vi "plot theory.vi"() -> ()   [LabVIEW 2016]
uses:
  <vilib>/Utility/file.llb/Write Delimited Spreadsheet (DBL).vi
panel:
  in  "color scale":u32[](array[colorbox])=[16711680, 16772608, 6618880, 3381759, 16860, 10420479]
  in  "length 2":i32=200
  in  "index 2":i32
  out "Intensity Graph 13":dbl[][](graph)
  in  "file path (dialog if empty)":path=path "C:/Users/ansom/OneDrive/Pascal Electron Bunching/Figures/Fig 4_new/DMRG stuff/trion_from labview.txt"
  out "Array 2":dbl[][](array[numeric])
  in  "DMRG #":i32=226
  in  "file (use dialog) 4":path=path "C:/Users/ansom/OneDrive/Pascal Electron Bunching/Figures/Fig 4_new/DMRG stuff/trion.txt"
  in  "length":i32=1000
  in  "index":i32
  out "input G":cluster{dbl[], dbl[]}[](graph)=[{[0.01, 0.02, 0.03, 0.04, 0.05, 0.060000000000000005, 0.06999999999999999, 0.08, 0.09, 0.09999999999999999, 0.11, 0.12, 0.13, 0.14, 0.15000000000000002, 0.16, 0.17, 0.18000000000000002, 0.19, 0.2, 0.21000000000000002, 0.22, 0.23, 0.24000000000000002, 0.25, 0.26, 0.27, 0.28, 0.29000000000000004, 0.3, 0.31, 0.32, 0.33, 0.34, 0.35000000000000003, 0.36000000000000004, 0.37, 0.38, 0.39, 0.4, 0.41000000000000003, 0.42000000000000004, 0.43, 0.44, 0.45, 0.46, 0.47000000000000003, 0.48000000000000004, 0.49, 0.5, 0.51, 0.52, 0.53, 0.54, 0.55, 0.56, 0.5700000000000001, 0.5800000000000001, 0.59, 0.6, 0.61, 0.62, 0.63, 0.64, 0.65, 0.66, 0.67, 0.68, 0.6900000000000001, 0.7000000000000001, 0.7100000000000001, 0.72, 0.73, 0.74, 0.75, 0.76, 0.77, 0.78, 0.79, 0.8, 0.81, 0.8200000000000001, 0.8300000000000001, 0.8400000000000001, 0.85, 0.86, 0.87, 0.88, 0.89, 0.9, 0.91, 0.92, 0.93, 0.9400000000000001, 0.9500000000000001, 0.9600000000000001, 0.97, 0.98, 0.99, 1.0, 1.01, 1.02, 1.03, 1.04, 1.05, 1.06, 1.07, 1.08, 1.09, 1.1, 1.11, 1.12, 1.1300000000000001, 1.1400000000000001, 1.1500000000000001, 1.1600000000000001, 1.17, 1.18, 1.19, 1.2, 1.21, 1.22, 1.23, 1.24, 1.25, 1.26, 1.27, 1.28, 1.29, 1.3, 1.31, 1.32, 1.33, 1.34, 1.35, 1.36, 1.37, 1.3800000000000001, 1.3900000000000001, 1.4000000000000001, 1.4100000000000001, 1.42, 1.43, 1.44, 1.45, 1.46, 1.47, 1.48, 1.49, 1.5, 1.51, 1.52, 1.53, 1.54, 1.55, 1.56, 1.57, 1.58, 1.59, 1.6, 1.61, 1.62, 1.6300000000000001, 1.6400000000000001, 1.6500000000000001, 1.6600000000000001, 1.6700000000000002, 1.68, 1.69, 1.7, 1.71, 1.72, 1.73, 1.74, 1.75, 1.76, 1.77, 1.78, 1.79, 1.8, 1.81, 1.82, 1.83, 1.84, 1.85, 1.86, 1.87, 1.8800000000000001, 1.8900000000000001, 1.9000000000000001, 1.9100000000000001, 1.9200000000000002, 1.93, 1.94, 1.95, 1.96, 1.97, 1.98, 1.99, 2.0], [0.0, 2.8179258963930954e-06, 5.865517131435599e-06, 1.1115444670828347e-05, 2.013415466013697e-05, 3.564578593329415e-05, 6.231356475073917e-05, 0.00010817567243315048, 0.0001870443462831501, 0.00032266888951518836, 0.0005559253396610961, 0.0009570334248864857, 0.0016466138487119166, 0.0028317168787741144, 0.004867094665031302, 0.008358909082529469, 0.014338061316041076, 0.02454336456201635, 0.04186555650718952, 0.07099477071552311, 0.1192181455270459, 0.19702751476009608, 0.31754465261583664, 0.4929918087827873, 0.7270707427374825, 1.0068315493607645, 1.303870994089269, 1.5898503592803936, 1.8542059202275674, 2.107927138772979, 2.372565955700939, 2.663658895477296, 2.978024236296329, 3.2945575894029333, 3.5907595763609583, 3.8607032966795023, 4.118417825912882, 4.386736502532661, 4.681005344958576, 4.997139339821397, 5.313617926593991, 5.608742028148086, 5.878098240348298, 6.136917865879712, 6.408381089034445, 6.707415756579491, 7.0295138846981375, 7.354050575014656, 7.662532325724841, 7.9559972758691035, 8.257068268102014, 8.59832499790761, 9.005858750273989, 9.485865728196863, 10.022010605260363, 10.585071760757913, 11.147313172231405, 11.695472331539898, 12.236800322485264, 12.79040913714259, 13.368853196684928, 13.96718630472856, 14.567363112985483, 15.15074818722707, 15.710997225632449, 16.26010468106789, 16.81951113752647, 17.40214872439687, 18.002767315246018, 18.60335954680593, 19.185992790268575, 19.745628904993918, 20.295452701683242, 20.85711245892441, 21.442832225062357, 22.046765008795422, 22.651313809011008, 23.240359487686586, 23.812234669482113, 24.38480624265897, 24.985518789665473, 25.634311044565536, 26.335976422740604, 27.085078807164205, 27.87323297330553, 28.692655259186335, 29.535612303041997, 30.392470291093304, 31.253112586227456, 32.11126213406538, 32.96669782438915, 33.823190913007124, 34.68503172743494, 35.55364233198232, 36.42553936546845, 37.29469772847206, 38.1576422255595, 39.015959727230076, 39.87442706067657, 40.73777794207555, 41.607477793911414, 42.479987901448624, 43.34947542419982, 44.21295855685387, 45.07258580489307, 45.9336602171978, 46.801526677239856, 47.67856262350638, 48.562979328968716, 49.452307104798635, 50.34919525380985, 51.264151190587604, 52.213679224779575, 53.21569295203033, 54.281404489557396, 55.40545289638095, 56.56294069425582, 57.72071321658015, 58.85736648074177, 59.97509976423845, 61.0945414605609, 62.237597573001054, 63.41005940897371, 64.59594439068273, 65.76911868877475, 66.9138986023004, 68.03666579771638, 69.16034526404309, 70.30725646245965, 71.48241599680148, 72.66905548648172, 73.8413370460884, 74.98496084644341, 76.1078700133423, 77.23376206365978, 78.38468495970822, 79.56489646936996, 80.75760780281024, 81.93892390590176, 83.09878006001364, 84.25127138493237, 85.4279730030069, 86.66068759066243, 87.96488912029083, 89.33334009472996, 90.74260884461259, 92.16574915118754, 93.58379408866665, 94.99404366324039, 96.40873804301812, 97.84163247726151, 99.29453862986917, 100.75605837577758, 102.21000947974164, 103.6457662539617, 105.06663578596623, 106.48846757504609, 107.92641937203824, 109.38245382309192, 110.84522457621912, 112.2989725664384, 113.7339654899229, 115.15460251908631, 116.57723208042141, 118.01649951245584, 119.47342872833094, 120.93610771377155, 122.38886223587953, 123.82265420342671, 125.24283755310711, 126.66611460936745, 128.1065090941953, 129.56404604963117, 131.02622118449602, 132.47737417640826, 133.9090314886612, 135.32721123994423, 136.7484139594865, 138.18516151830661, 139.63509629879908, 141.08280857857633, 142.50881111150676, 143.89904436452576, 145.2507726450103, 146.567316973192, 147.8447583157048, 149.06680014188356, 150.21556039701025, 151.28537528193894, 152.2847286798789, 153.22664057547803, 154.11777948305541, 154.9551366322349, 155.72976866205235, 156.43200642589352, 157.05608678065863, 157.60563194109096, 158.09445966431034, 158.53561617308696, 158.92790708641883]}, ...(100 in all)]
  in  "mu":path=path "C:/Users/ansom/OneDrive/Pascal Electron Bunching/Figures/Fig 3_new/mathematica/mu.txt"
  in  "G":path=path "C:/Users/ansom/OneDrive/Pascal Electron Bunching/Figures/Fig 3_new/mathematica/Gsteps_g=1"
  in  "Numeric 2":i32=100
  in  "Numeric":i32=360
  out "Intensity Graph 12":dbl[][](graph)
  out "Array":dbl[][](array[numeric])
  in  "file (use dialog)":path=path "C:/Users/ansom/OneDrive/Pascal Electron Bunching/Figures/Fig 3_new/mathematica/ModeldGdE"
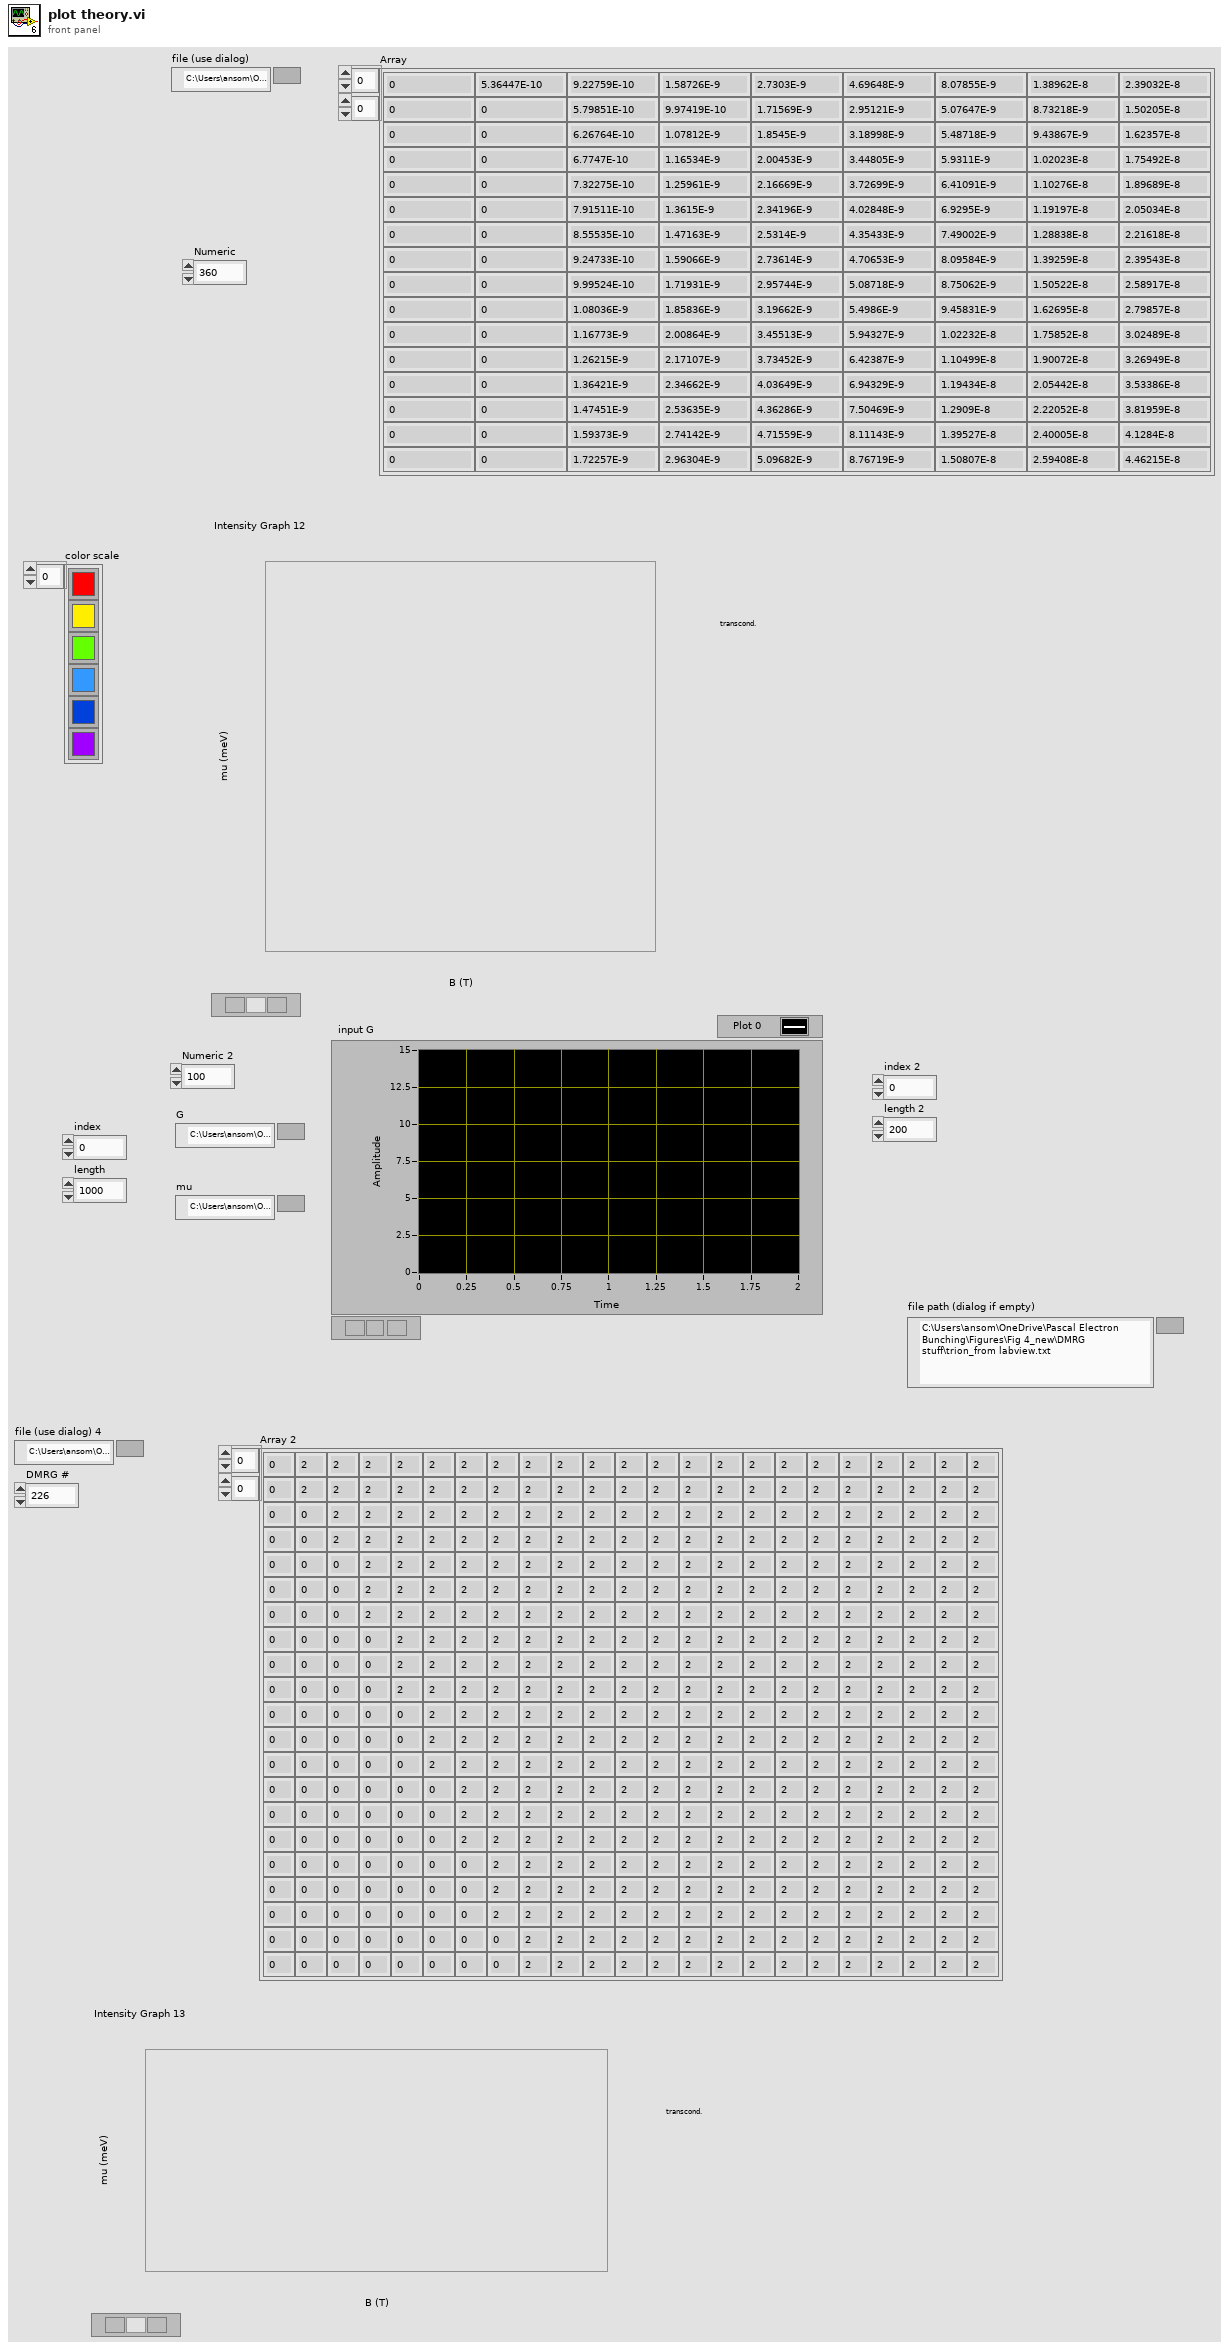
[diagram p1: front panel]
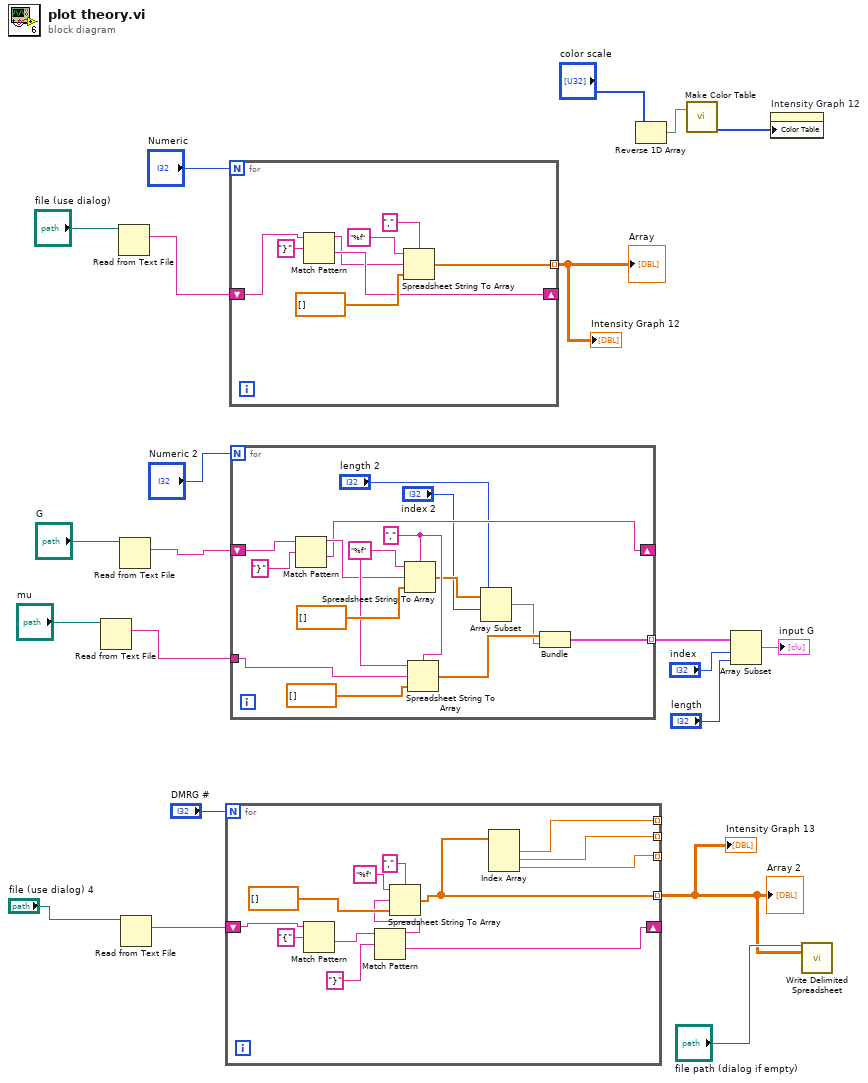
[diagram p0: block diagram]
diagram:
  n1 = Read from Text File(file (use dialog)="mu") -> (text=w14:string)  [unwired: 3 in, 3 out]
  n2 = Read from Text File(file (use dialog)="file (use dialog)") -> (text=w20:string)  [unwired: 3 in, 3 out]
  n3 = Read from Text File(file (use dialog)="G") -> (text=w13:string)  [unwired: 3 in, 3 out]
  n4 = Read from Text File(file (use dialog)="file (use dialog) 4") -> (text=w7:string)  [unwired: 3 in, 3 out]
  n5 = for {
    N: "DMRG #" -> [_]
    shift-right: [w26] -> _
    shift-left: w7 -> [w33]
    tunnel: [w25] -> w4 mode=indexing
    tunnel: [w24] -> _ mode=indexing
    tunnel: [w23] -> _ mode=indexing
    tunnel: [w22] -> _ mode=indexing
    n6 = Match Pattern(string=w33, regular expression="{") -> (after substring=w29:string)  [unwired: 1 in, 3 out]
    n7 = Match Pattern(string=w29, regular expression="}") -> (before substring=w27:string, after substring=w26:string)  [unwired: 1 in, 2 out]
    n8 = Spreadsheet String To Array(delimiter (Tab)=",", format string="%f", spreadsheet string=w27, array type (2D Dbl)=dbl[] []) -> (array=w25:dbl[])
    n9 = Index Array(array=w25) -> (element #1=w24:dbl, element #2=w23:dbl, element #3=w22:dbl)  [unwired: 3 in]
  }
  "Array 2" <- w4
  "Intensity Graph 13" <- w4
  n10 = for {
    N: "Numeric" -> [_]
    tunnel: [w38] -> w18 mode=indexing
    shift-right: [w37] -> _
    shift-left: w20 -> [w36]
    n11 = Match Pattern(string=w36, regular expression="}") -> (before substring=w35:string, after substring=w37:string)  [unwired: 1 in, 2 out]
    n12 = Spreadsheet String To Array(delimiter (Tab)=",", format string="%f", spreadsheet string=w35, array type (2D Dbl)=dbl[] []) -> (array=w38:dbl[])
  }
  "Array" <- w18
  "Intensity Graph 12" <- w18
  n13 = for {
    N: "Numeric 2" -> [_]
    tunnel: w14 -> [w56]
    tunnel: [w52] -> w12 mode=indexing
    shift-right: [w48] -> _
    shift-left: w13 -> [w51]
    w55 = "%f" ("format string")
    w54 = "," ("delimiter (Tab)")
    n14 = Match Pattern(string=w51, regular expression="}") -> (before substring=w49:string, after substring=w48:string)  [unwired: 1 in, 2 out]
    n15 = Spreadsheet String To Array(delimiter (Tab)=w54, format string=w55, spreadsheet string=w49, array type (2D Dbl)=dbl[] []) -> (array=w46:dbl[])
    n16 = Spreadsheet String To Array(delimiter (Tab)=w54, format string=w55, spreadsheet string=w56, array type (2D Dbl)=dbl[] []) -> (array=w47:dbl[])
    n17 = Array Subset(array=w46, index="index 2", length="length 2") -> (w45:dbl[])
    n18 = Bundle(w47, w45) -> (w52:cluster{dbl[], dbl[]})  [unwired: 1 in]
  }
  n19 = Reverse 1D Array(array="color scale") -> (reversed array=w2:u32[])
  n20 = call <userlib>:"Make Color Table.vi"("Array"=w2) -> ("Color Tbl"=w3:u32[])  [unwired: 1 in, 3 out]
  n21 = Array Subset(array=w12, index="index", length="length") -> (→"input G":cluster{dbl[], dbl[]}[])
  n22 = property on="Intensity Graph 12" class="IntGraph (strict)"("Color Table"=w3) -> ()  [unwired: 2 in, 2 out]
  n23 = call-poly <vilib>:"Write Delimited Spreadsheet.vi"("file path (dialog if empty)"="file path (dialog if empty)", "2D data"=w4) -> ()  [unwired: 12 in, 2 out]
